vi "诊断标定3.vi"(8 "CAN端口":u16(ring), 9 "设备索引号":u16(ring), 10 "CAN卡类型":u32(ring)=21) -> ()   [LabVIEW 2013] (continued)
                                n480 = call "表格编辑(版本读取).vi"("新元素/子数组"=w689, "活动单元格:单元格背景色"=u32 6618880, "MCListbox引用句柄"=w690) -> ()  [unwired: 1 in, 8 out]
                                }
                                frame 3 {
                                n481 = Index Array(array=w720, index #1=0 ("索引"), index #2=1 ("索引")) -> (element #1=w716:u8, element #2=w717:u8)
                                n482 = Join Numbers(hi=w716, lo=w717) -> ((hi.lo)=w715:u16)
                                n483 = case shown="99, 默认" w715 {
                                tunnel: w720 -> [w723 _ w757]
                                tunnel: w715 -> [_ _ w735]
                                frame 0 {
                                n484 = Index Array(array=w723, index #1=2 ("索引"), index #2=3 ("索引")) -> (element #1=w727:u8, element #2=w726:u8)
                                n485 = Join Numbers(hi=w727, lo=w726) -> ((hi.lo)=w722:u16)
                                n486 = for {
                                N: w722 -> [_]
                                tunnel: w723 -> [w732]
                                tunnel: [w728] -> w721 mode=indexing
                                i -> [w731]
                                n487 = Add(x=w731, y=4) -> (x+y=w729:i32)
                                n488 = Index Array(array=w732, index=w729) -> (element=w728:u8)
                                }
                                "MODEL号" <- w721
                                }
                                frame 99, Default {
                                }
                                frame 1..40 {
                                w740 = ""
                                w761 = "." ("字符串")
                                n489 = Array Subset(array=w757, index=2 ("索引"), length=14 ("长度")) -> (w746:u8[])
                                n490 = Index Array(array=w757, index=16 ("索引")) -> (element=w769:u8)
                                n491 = Index Array(array=w757, index #1=17 ("索引"), index #2=18 ("索引")) -> (element #1=w775:u8, element #2=w776:u8)
                                n492 = Index Array(array=w757, index #1=19 ("索引"), index #2=20 ("索引")) -> (element #1=w770:u8, element #2=w771:u8)
                                n493 = Join Numbers(hi=w770, lo=w771) -> ((hi.lo)=w767:u16)
                                n494 = Join Numbers(hi=w775, lo=w776) -> ((hi.lo)=w768:u16)
                                n495 = Number To Decimal String(number=w735) -> (decimal integer string=w755:string)  [unwired: 1 out]
                                n496 = Number To Decimal String(number=w769) -> (decimal integer string=w763:string)  [unwired: 1 out]
                                n497 = call "数组去零.vi"("输入"=w746) -> ("输出"=w745:dbl[])
                                n498 = Number To Decimal String(number=w768) -> (decimal integer string=w762:string)  [unwired: 1 out]
                                n499 = Number To Decimal String(number=w767) -> (decimal integer string=w760:string)  [unwired: 1 out]
                                n500 = Byte Array To String(unsigned byte array=w745) -> (string=w747:string)
                                n501 = Concatenate Strings("第" ("读取结果"), w755, "模块" ("字符串"), "     读取完成" ("读取结果")) -> (w748:string)
                                n502 = Concatenate Strings("V" ("字符串"), w763, w761, w762, w761, w760) -> (w758:string)
                                n503 = control-ref of="结果"() -> (w751:refnum<vi>)
                                n504 = Array Subset(array=w757, index=23 ("索引"), length=7 ("长度")) -> (w744:u8[])
                                n505 = call "数组去零.vi"("输入"=w744) -> ("输出"=w739:dbl[])
                                n506 = Byte Array To String(unsigned byte array=w739) -> (string=w736:string)
                                n507 = Build Array(w748) -> (w750:string[])
                                n508 = control-ref of="模块软件版本 2"() -> (w752:refnum<vi>)
                                n509 = local read "模块软件版本"() -> (w753:T1)
                                n510 = Equal?(x=w740, y=w736) -> (x = y?=w741:bool)
                                n511 = call "表格编辑(版本读取).vi"("新元素/子数组"=w750, "活动单元格:单元格背景色"=u32 6618880, "MCListbox引用句柄"=w751) -> ()  [unwired: 1 in, 8 out]
                                n512 = Concatenate Strings("-" ("字符串"), w736) -> (w742:string)
                                n513 = Select(t=w740, s=w741, f=w742) -> (s? t:f=w738:string)
                                n514 = Concatenate Strings(w747, "-" ("字符串"), w758, w738) -> (w737:string)
                                n515 = case shown="30" w735 {
                                tunnel: [_ "VERSIONM" "BCUMCAL" "BMUMCAL" "BMURMCAL" "BCUCMCAL" "BCUDMCAL" "SCH" "BSW" "CDD" "DATALAYER" "DATAANALYSIS" "SOC" "SOH" "SOF" "INTRES" "INTCAN" "CARCAN" "CHGCANL" "THM" "CHGM" "HVM" "LVM" "BALM" "SAFEM" "RUNMODEM" "RELAY" "DO" "GBCHGDET" "SUPPLYPOWGDET" "SUMVDET" "CURDET" "TEMPERDET" "CELLVDET" "ISODET" "AI" "DI" "SYSCONF" "ECUCONF"] -> w734
                                frame 0, Default {
                                }
                                frame 1 {
                                }
                                frame 2 {
                                }
                                frame 3 {
                                }
                                frame 4 {
                                }
                                frame 5 {
                                }
                                frame 6 {
                                }
                                frame 7 {
                                }
                                frame 8 {
                                }
                                frame 9 {
                                }
                                frame 10 {
                                }
                                frame 11 {
                                }
                                frame 12 {
                                }
                                frame 13 {
                                }
                                frame 14 {
                                }
                                frame 15 {
                                }
                                frame 16 {
                                }
                                frame 17 {
                                }
                                frame 18 {
                                }
                                frame 19 {
                                }
                                frame 20 {
                                }
                                frame 21 {
                                }
                                frame 22 {
                                }
                                frame 23 {
                                }
                                frame 24 {
                                }
                                frame 25 {
                                }
                                frame 26 {
                                }
                                frame 27 {
                                }
                                frame 28 {
                                }
                                frame 29 {
                                }
                                frame 30 {
                                }
                                frame 31 {
                                }
                                frame 32 {
                                }
                                frame 33 {
                                }
                                frame 34 {
                                }
                                frame 35 {
                                }
                                frame 36 {
                                }
                                frame 37 {
                                }
                                frame 38 {
                                }
                                }
                                n516 = case shown="\"全部读取\"" w753 {
                                tunnel: w737 -> [w820 w828]
                                tunnel: w735 -> [w824 w833]
                                tunnel: w752 -> [w826 w834]
                                tunnel: w734 -> [w825 w832]
                                frame "全部读取" {
                                n517 = Number To Decimal String(number=w824) -> (decimal integer string=w823:string)  [unwired: 1 out]
                                n518 = Concatenate Strings(w823, "-" ("元素"), w825) -> (w821:string)
                                n519 = Build Array(w821, w820) -> (w819:string[])
                                n520 = call "表格编辑(模块版本).vi"("新元素/子数组"=w819, "MCListbox引用句柄"=w826) -> ()  [unwired: 1 in, 9 out]
                                }
                                frame "BCUMCAL", Default {
                                n521 = Number To Decimal String(number=w833) -> (decimal integer string=w831:string)  [unwired: 1 out]
                                n522 = Concatenate Strings(w831, "-" ("元素"), w832) -> (w829:string)
                                n523 = Build Array(w829, w828) -> (w827:string[])
                                n524 = call "表格编辑(模块版本).vi"("新元素/子数组"=w827, "MCListbox引用句柄"=w834) -> ()  [unwired: 1 in, 9 out]
                                }
                                }
                                }
                                }
                                }
                                frame 4 {
                                n525 = Array Subset(array=w847, length=12 ("长度")) -> (w845:u8[])  [unwired: 1 in]
                                n526 = Byte Array To String(unsigned byte array=w845) -> (string=w844:string)
                                n527 = call <vilib>:"Trim Whitespace.vi"("string"=w844) -> ("trimmed string"=w836:string)  [unwired: 1 in]
                                n528 = local read "从板板号"() -> (w835:u8)
                                n529 = local write "硬件版本号"(w836) -> ()
                                n530 = local read "硬件版本"() -> (w837:string[])
                                n531 = Replace Array Subset(array=w837, new element=w836, index=w835) -> (w838:string[])
                                n532 = local write "硬件版本"(w838) -> ()
                                n533 = global write "EV05全局变量1.vi" "写入超时"(TRUE ("写入超时")) -> ()
                                n534 = control-ref of="结果"() -> (w842:refnum<vi>)
                                n535 = Build Array("硬件版本     读取完成" ("读取结果")) -> (w841:string[])
                                n536 = call "表格编辑(版本读取).vi"("新元素/子数组"=w841, "活动单元格:单元格背景色"=u32 6618880, "MCListbox引用句柄"=w842) -> ()  [unwired: 9 out]
                                }
                              }
                              n537 = global write "EV05全局变量1.vi" "写入超时"(TRUE ("写入超时")) -> ()
                            }
                          }
                        }
                        frame True {
                          n538 = Index Array(array=w849, index #1=0 ("索引"), index #2=1 ("索引")) -> (element #1=w854:u8, element #2=w855:u8)
                          n539 = Join Numbers(hi=w854, lo=w855) -> ((hi.lo)=w853:u16)
                          n540 = Number To Hexadecimal String(2:w853) -> (0:w852:string)  [unwired: 1 out]
                          n541 = control-ref of="结果"() -> (w851:refnum<vi>)
                          n542 = Concatenate Strings("0x" ("字符串"), w852) -> (w859:string)
                          n543 = Build Array(w859) -> (w850:string[])
                          n544 = call "表格编辑(版本读取).vi"("新元素/子数组"=w850, "活动单元格:单元格背景色"=u32 16740749, "MCListbox引用句柄"=w851) -> ()  [unwired: 9 out]
                        }
                      }
                      n545 = global write "EV05全局变量1.vi" "流控帧 2"(FALSE ("流控帧 2")) -> ()
                      n546 = local write "控制1"(FALSE ("控制1")) -> ()
                      n547 = local write "消除"(FALSE ("消除")) -> ()
                      n548 = call <vilib>:"Unset Busy.vi"() -> ()  [unwired: 2 in, 10 out]
                    }
                  }
                }
                frame "其它诊断" {
                  n549 = local read "命令序号"() -> (w861:u8)
                  n550 = call "多帧接收机制(EV05).vi"("can卡类型"=w868, "设备索引号"=w867, "CAN端口"=w866, "VCI_Receive"=w865, "命令"=w863, "板号"=w864, "命令序号"=w861) -> ("错误代码"=w870:i32, "输出数组"=w862:u8[], "读错误代码"=w860:u8[], "结束信号"=w869:bool)  [unwired: 1 in, 8 out]
                  n551 = case shown="真" w869 {
                    tunnel: w871 -> [_ w872]
                    tunnel: w870 -> [_ _]
                    tunnel: w862 -> [_ w873]
                    tunnel: w861 -> [_ w876]
                    tunnel: w860 -> [_ w874]
                    frame False {
                    }
                    frame True {
                      n552 = Insert Into Array(array=w874, new element=w873) -> (w875:u8[])  [unwired: 1 in]
                      n553 = case shown="1" w876 {
                        tunnel: w875 -> [_ w885 w971]
                        tunnel: w872 -> [_ _ w966]
                        frame 0, Default {
                        }
                        frame 1 {
                          n554 = Index Array(array=w885) -> (element #1=w884:u8, element #2=w883:u8, element #3=w882:u8)  [unwired: 3 in]
                          n555 = Join Numbers(hi=w883, lo=w882) -> ((hi.lo)=w881:u16)
                          n556 = case shown="4" w884 {
                            tunnel: w885 -> [_ _ _ _ _ _ _ _ _ _]
                            tunnel: w881 -> [_ w888 w896 w906 w916 w926 w936 w946 w956 _]
                            frame 0, Default {
                              n557 = local write "继电器超时处理"(FALSE ("继电器超时处理")) -> ()
                            }
                            frame 1 {
                              n558 = Equal To 0?(x=w888) -> (x = 0?=w887:bool)
                              n559 = local write "正级继电器 12"(w887) -> ()
                              n560 = case shown="假" w887 {
                                tunnel: w888 -> [w891 _]
                                frame False {
                                n561 = local read "正级继电器"() -> (w893:bool)
                                n562 = Number To Hexadecimal String(2:w891) -> (0:w890:string)  [unwired: 1 out]
                                n563 = local write "继电器超时处理"(TRUE ("继电器超时处理")) -> ()
                                n564 = Not(x=w893) -> (.not. x?=w892:bool)
                                n565 = Concatenate Strings("继电器操作失败,0x" ("消息"), w890) -> ()  [unwired: 1 out]
                                n566 = local write "正级继电器"(w892) -> ()
                                }
                                frame True {
                                (unwired) "继电器操作成功!\n继电器操作成功!\n继电器操作成功!"
                                }
                              }
                            }
                            frame 2 {
                              n567 = Equal To 0?(x=w896) -> (x = 0?=w895:bool)
                              n568 = case shown="假" w895 {
                                tunnel: w896 -> [w902 _]
                                tunnel: [w900 "继电器操作成功!\n继电器操作成功!\n继电器操作成功!"] -> _
                                frame False {
                                n569 = local read "负级继电器"() -> (w898:bool)
                                n570 = Number To Hexadecimal String(2:w902) -> (0:w901:string)  [unwired: 1 out]
                                n571 = local write "继电器超时处理"(TRUE ("继电器超时处理")) -> ()
                                n572 = Not(x=w898) -> (.not. x?=w899:bool)
                                n573 = Concatenate Strings("继电器操作失败,0x" ("消息"), w901) -> (w900:string)
                                n574 = local write "负级继电器"(w899) -> ()
                                }
                                frame True {
                                }
                              }
                              n575 = local write "正级继电器 2"(w895) -> ()
                            }
                            frame 3 {
                              n576 = Equal To 0?(x=w906) -> (x = 0?=w905:bool)
                              n577 = case shown="假" w905 {
                                tunnel: w906 -> [w912 _]
                                tunnel: [w910 "继电器操作成功!\n继电器操作成功!\n继电器操作成功!"] -> _
                                frame False {
                                n578 = local read "预充电继电器"() -> (w908:bool)
                                n579 = Number To Hexadecimal String(2:w912) -> (0:w911:string)  [unwired: 1 out]
                                n580 = local write "继电器超时处理"(TRUE ("继电器超时处理")) -> ()
                                n581 = Not(x=w908) -> (.not. x?=w909:bool)
                                n582 = Concatenate Strings("继电器操作失败,0x" ("消息"), w911) -> (w910:string)
                                n583 = local write "预充电继电器"(w909) -> ()
                                }
                                frame True {
                                }
                              }
                              n584 = local write "正级继电器 3"(w905) -> ()
                            }
                            frame 4 {
                              n585 = Equal To 0?(x=w916) -> (x = 0?=w915:bool)
                              n586 = case shown="假" w915 {
                                tunnel: w916 -> [w922 _]
                                tunnel: [w920 "继电器操作成功!\n继电器操作成功!\n继电器操作成功!"] -> _
                                frame False {
                                n587 = local read "加热继电器"() -> (w919:bool)
                                n588 = Number To Hexadecimal String(2:w922) -> (0:w921:string)  [unwired: 1 out]
                                n589 = local write "继电器超时处理"(TRUE ("继电器超时处理")) -> ()
                                n590 = Not(x=w919) -> (.not. x?=w918:bool)
                                n591 = Concatenate Strings("继电器操作失败,0x" ("消息"), w921) -> (w920:string)
                                n592 = local write "加热继电器"(w918) -> ()
                                }
                                frame True {
                                }
                              }
                              n593 = local write "正级继电器 5"(w915) -> ()
                            }
                            frame 5 {
                              n594 = Equal To 0?(x=w926) -> (x = 0?=w925:bool)
                              n595 = case shown="假" w925 {
                                tunnel: w926 -> [w932 _]
                                tunnel: [w930 "继电器操作成功!\n继电器操作成功!\n继电器操作成功!"] -> _
                                frame False {
                                n596 = local read "充电继电器"() -> (w928:bool)
                                n597 = Number To Hexadecimal String(2:w932) -> (0:w931:string)  [unwired: 1 out]
                                n598 = local write "继电器超时处理"(TRUE ("继电器超时处理")) -> ()
                                n599 = Not(x=w928) -> (.not. x?=w929:bool)
                                n600 = Concatenate Strings("继电器操作失败,0x" ("消息"), w931) -> (w930:string)
                                n601 = local write "充电继电器"(w929) -> ()
                                }
                                frame True {
                                }
                              }
                              n602 = local write "正级继电器 4"(w925) -> ()
                            }
                            frame 6 {
                              n603 = Equal To 0?(x=w936) -> (x = 0?=w935:bool)
                              n604 = local write "正级继电器 6"(w935) -> ()
                              n605 = case shown="假" w935 {
                                tunnel: w936 -> [w942 _]
                                tunnel: [w940 "继电器操作成功!\n继电器操作成功!\n继电器操作成功!"] -> _
                                frame False {
                                n606 = local read "风机继电器"() -> (w938:bool)
                                n607 = Number To Hexadecimal String(2:w942) -> (0:w941:string)  [unwired: 1 out]
                                n608 = local write "继电器超时处理"(TRUE ("继电器超时处理")) -> ()
                                n609 = Not(x=w938) -> (.not. x?=w939:bool)
                                n610 = Concatenate Strings("继电器操作失败,0x" ("消息"), w941) -> (w940:string)
                                n611 = local write "风机继电器"(w939) -> ()
                                }
                                frame True {
                                }
                              }
                            }
                            frame 7 {
                              n612 = Equal To 0?(x=w946) -> (x = 0?=w945:bool)
                              n613 = case shown="假" w945 {
                                tunnel: w946 -> [w951 _]
                                tunnel: [w949 "继电器操作成功!\n继电器操作成功!\n继电器操作成功!"] -> _
                                frame False {
                                n614 = local read "加热继电器(从)"() -> (w947:bool)
                                n615 = Number To Hexadecimal String(2:w951) -> (0:w950:string)  [unwired: 1 out]
                                n616 = Not(x=w947) -> (.not. x?=w948:bool)
                                n617 = Concatenate Strings("继电器操作失败,0x" ("消息"), w950) -> (w949:string)
                                n618 = local write "加热继电器(从)"(w948) -> ()
                                }
                                frame True {
                                n619 = local write "继电器超时处理"(TRUE ("继电器超时处理")) -> ()
                                }
                              }
                              n620 = local write "正级继电器 7"(w945) -> ()
                            }
                            frame 8 {
                              n621 = Equal To 0?(x=w956) -> (x = 0?=w955:bool)
                              n622 = case shown="假" w955 {
                                tunnel: w956 -> [w961 _]
                                tunnel: [w959 "继电器操作成功!\n继电器操作成功!\n继电器操作成功!"] -> _
                                frame False {
                                n623 = local read "风机继电器(从)"() -> (w957:bool)
                                n624 = Number To Hexadecimal String(2:w961) -> (0:w960:string)  [unwired: 1 out]
                                n625 = Not(x=w957) -> (.not. x?=w958:bool)
                                n626 = Concatenate Strings("继电器操作失败,0x" ("消息"), w960) -> (w959:string)
                                n627 = local write "风机继电器(从)"(w958) -> ()
                                }
                                frame True {
                                n628 = local write "继电器超时处理"(TRUE ("继电器超时处理")) -> ()
                                }
                              }
                              n629 = local write "正级继电器 8"(w955) -> ()
                            }
                            frame 85, 170 {
                              n630 = local write "继电器超时处理"(TRUE ("继电器超时处理")) -> ()
                            }
                          }
                        }
                        frame 2 {
                          n631 = Index Array(array=w971) -> (element #1=w970:u8, element #2=w969:u8, element #3=w968:u8)  [unwired: 3 in]
                          n632 = Join Numbers(hi=w969, lo=w968) -> ((hi.lo)=w967:u16)
                          n633 = case shown="2" w970 {
                            tunnel: w971 -> [_ _ _]
                            tunnel: w967 -> [_ w975 w989]
                            tunnel: w966 -> [_ w974 _]
                            frame 0, Default {
                              n634 = local write "继电器超时处理"(FALSE ("继电器超时处理")) -> ()
                            }
                            frame 1 {
                              n635 = Equal To 0?(x=w975) -> (x = 0?=w973:bool)
                              n636 = case shown="假" w973 {
                                tunnel: w975 -> [w981 _]
                                tunnel: [w979 "DO控制操作成功!\nDO控制操作成功!\nDO控制操作成功!"] -> _
                                tunnel: w974 -> [w978 _]
                                frame False {
                                n637 = case shown="\"主板\", 默认" w978 {
                                frame "主板", Default {
                                n638 = local read "DO1"() -> (w984:bool)
                                n639 = Not(x=w984) -> (.not. x?=w983:bool)
                                n640 = local write "DO1"(w983) -> ()
                                }
                                frame "从板" {
                                n641 = local read "DO1 2"() -> (w986:bool)
                                n642 = Not(x=w986) -> (.not. x?=w985:bool)
                                n643 = local write "DO1 2"(w985) -> ()
                                }
                                }
                                n644 = Number To Hexadecimal String(2:w981) -> (0:w980:string)  [unwired: 1 out]
                                n645 = Concatenate Strings("DO控制操作失败,0x" ("消息"), w980) -> (w979:string)
                                }
                                frame True {
                                }
                              }
                              n646 = case shown="\"从板\"" w974 {
                                tunnel: w973 -> [w976 w977]
                                frame "主板", Default {
                                n647 = local write "正级继电器 9"(w976) -> ()
                                }
                                frame "从板" {
                                n648 = local write "正级继电器 11"(w977) -> ()
                                }
                              }
                            }
                            frame 2 {
                              n649 = Equal To 0?(x=w989) -> (x = 0?=w988:bool)
                              n650 = case shown="假" w988 {
                                tunnel: w989 -> [w994 _]
                                tunnel: [w992 "DO控制操作成功!\nDO控制操作成功!\nDO控制操作成功!"] -> _
                                frame False {
                                n651 = Number To Hexadecimal String(2:w994) -> (0:w993:string)  [unwired: 1 out]
                                n652 = local read "DO2"() -> (w991:bool)
                                n653 = Not(x=w991) -> (.not. x?=w990:bool)
                                n654 = Concatenate Strings("DO控制操作失败,0x" ("消息"), w993) -> (w992:string)
                                n655 = local write "DO2"(w990) -> ()
                                }
                                frame True {
                                }
                              }
                              n656 = local write "正级继电器 10"(w988) -> ()
                            }
                          }
                        }
                      }
                      n657 = local write "消除"(FALSE ("消除")) -> ()
                      n658 = global write "EV05全局变量1.vi" "流控帧 2"(FALSE ("流控帧 2")) -> ()
                      n659 = local write "控制1"(FALSE ("控制1")) -> ()
                      "继电器超时处理" <- TRUE ("控制1")
                    }
                  }
                }
                frame "高压板校正" {
                  n660 = local read "命令序号"() -> (w1001:u8)
                  n661 = call "多帧接收机制(EV05).vi"("can卡类型"=w1008, "设备索引号"=w1007, "CAN端口"=w1006, "VCI_Receive"=w1005, "命令"=w1003, "板号"=w1004, "命令序号"=w1001) -> ("错误信号"=w997:bool, "错误代码"=w1010:i32, "输出数组"=w1002:u8[], "读错误代码"=w1000:u8[], "结束信号"=w1009:bool)  [unwired: 1 in, 7 out]
                  n662 = local read "控制1"() -> (w998:bool)
                  n663 = And(x=w998, y=w1009) -> (x .and. y?=w999:bool)
                  n664 = case shown="真" w999 {
                    tunnel: w1011 -> [_ w1015]
                    tunnel: w1010 -> [_ _]
                    tunnel: w1002 -> [_ w1013]
                    tunnel: w1001 -> [_ w1014]
                    tunnel: w1000 -> [_ w1016]
                    tunnel: w997 -> [_ w1017]
                    frame False {
                    }
                    frame True {
                      n665 = case shown="假" w1017 {
                        tunnel: w1016 -> [_ w1227]
                        tunnel: w1015 -> [_ _]
                        tunnel: w1014 -> [w1022 _]
                        tunnel: w1013 -> [w1021 _]
                        frame False {
                          n666 = case shown="2" w1022 {
                            tunnel: w1021 -> [_ w1027 w1061 w1091 w1118 w1145 w1172 w1199]
                            frame 0, Default {
                            }
                            frame 1 {
                              n667 = for {
                                N: 10 -> [_]
                                tunnel: w1027 -> [w1044]
                                shift-right: [w1031] -> w1025
                                shift-left: string[] [] -> [w1033]
                                i -> [w1030]
                                w1038 = 8 ("索引")
                                w1042 = 2 ("y")
                                n668 = Multiply(x=w1030, y=w1042) -> (x*y=w1043:i32)
                                n669 = Array Subset(array=w1044, index=w1043, length=w1042) -> (w1041:u8[])
                                n670 = Index Array(array=w1041) -> (element #1=w1040:u8, element #2=w1039:u8)  [unwired: 2 in]
                                n671 = call "二进制解析-8.6.vi"("索引"=w1038, "数值"=w1040) -> ("低位子数组"=w1037:i32[])  [unwired: 1 in, 2 out]
                                n672 = call "二进制解析-8.6.vi"("索引"=w1038, "数值"=w1039) -> ("低位子数组"=w1036:i32[])  [unwired: 1 in, 2 out]
                                n673 = Insert Into Array(array=w1037, new element=w1036) -> (w1035:i32[])  [unwired: 1 in]
                                n674 = case shown="2" w1030 {
                                tunnel: [6 15 9 4 2 0 2] -> w1029
                                frame 0, Default {
                                }
                                frame 1 {
                                }
                                frame 2 {
                                }
                                frame 3..5 {
                                }
                                frame 8, 9 {
                                }
                                frame 7 {
                                }
                                frame 6 {
                                }
                                }
                                n675 = Reverse 1D Array(array=w1035) -> (reversed array=w1034:i32[])
                                n676 = for {
                                N: w1029 -> [_]
                                tunnel: w1034 -> [w1056] mode=indexing
                                tunnel: [w1052] -> w1032 mode=indexing
                                n677 = Equal To 0?(x=w1056) -> (x = 0?=w1055:bool)
                                n678 = Select(t="无", s=w1055, f="故障") -> (s? t:f=w1052:string)
                                }
                                n679 = Insert Into Array(array=w1033, new element=w1032) -> (w1031:string[])  [unwired: 1 in]
                              }
                              n680 = call "详细故障分解.vi"("名称"=string[] ["上电自检异常(CellV)", "通讯异常(CellV)", "不更新(CellV)", "未校准(CellV)", "保留", "采样线路断路(CellV)", "18b20上电自检异常(T) ", "18b20通讯异常(T)", "18b20传感器丢失(T)", "18b20传感器无号(T)", "18b20温度异常跳变(T)", "18b20信号线对电源短路(T)", "18b20信号线对地短路(T)", "18b20 CRC校验异常(T)", "NTC上电自检异常(T)", "NTC通讯异常(T)", "NTC传感器丢失(T)", "NTC温度异常跳变(T)", "NTC信号线断路(T)", "NTC信号线对电源短(T)", "NTC信号线对地短路(T)", "上电自检异常(Curr)", "参数异常(Curr)", "不更新(Curr)", "未校准(Curr)", "采样线断开(Curr)", "电流零漂异常(Curr)", "传感器反接(Curr)", "读取实时电流故障(Curr)", "平均电流故障(Curr)", "自检异常(iso)", "前端检测电阻损坏(iso)", "不更新(iso)", "未校准(iso)", "上电自检异常(Sumv_in)", "通讯异常(Sumv_in)", "不更新(Sumv_in)", "未校准(Sumv_in)", "上电自检异常(Sumv_out)", "通讯异常(Sumv_out)", "不更新(Sumv_out)", "未校准(Sumv_out)", "系统时钟自检异常(Clock)", "系统时钟未校准(Clock)", "充电均衡模块不能开启", "充电均衡模块不能关闭", "放电均衡模块不能开启", "放电均衡模块不能关闭"], "故障输入口"=w1025) -> ("输出数组"=w1023:string[][])  [unwired: 1 in, 2 out]
                              n681 = local write "电池故障"(w1023) -> ()
                            }
                            frame 2 {
                              n682 = for {
                                N: 5 -> [_]
                                tunnel: w1061 -> [w1078]
                                shift-right: [w1065] -> w1059
                                shift-left: string[] [] -> [w1067]
                                i -> [w1063]
                                w1072 = 8 ("索引")
                                w1076 = 2 ("y")
                                n683 = Multiply(x=w1063, y=w1076) -> (x*y=w1077:i32)
                                n684 = Array Subset(array=w1078, index=w1077, length=w1076) -> (w1075:u8[])
                                n685 = Index Array(array=w1075) -> (element #1=w1074:u8, element #2=w1073:u8)  [unwired: 2 in]
                                n686 = call "二进制解析-8.6.vi"("索引"=w1072, "数值"=w1074) -> ("低位子数组"=w1071:i32[])  [unwired: 1 in, 2 out]
                                n687 = call "二进制解析-8.6.vi"("索引"=w1072, "数值"=w1073) -> ("低位子数组"=w1070:i32[])  [unwired: 1 in, 2 out]
                                n688 = Insert Into Array(array=w1071, new element=w1070) -> (w1069:i32[])  [unwired: 1 in]
                                n689 = case shown="2" w1063 {
                                tunnel: [4 6 5] -> w1064
                                frame 0, Default {
                                }
                                frame 2 {
                                }
                                frame 4 {
                                }
                                }
                                n690 = Reverse 1D Array(array=w1069) -> (reversed array=w1068:i32[])
                                n691 = for {
                                N: w1064 -> [_]
                                tunnel: w1068 -> [w1086] mode=indexing
                                tunnel: [w1082] -> w1066 mode=indexing
                                n692 = Equal To 0?(x=w1086) -> (x = 0?=w1085:bool)
                                n693 = Select(t="无", s=w1085, f="故障") -> (s? t:f=w1082:string)
                                }
                                n694 = Insert Into Array(array=w1067, new element=w1066) -> (w1065:string[])  [unwired: 1 in]
                              }
                              n695 = call "详细故障分解.vi"("名称"=string[] ["自检异常(ee_cpu)", "存储空间满(ee_cpu)", "数据写入失败(ee_cpu)", "数据读取异常(ee_cpu)", "自检异常(ee_ext)", "存储空间满(ee_ext)", "数据写入失败(ee_ext)", "数据读取异常(ee_ext)", "自检异常(flash_ext)", "故障数据存储空间满(flash_ext)", "历史数据存储空间满(flash_ext)", "数据写入失败(flash_ext)", "数据读取失败(flash_ext)", "数据校验异常(flash_ext)", "自检异常(flash_cpu)", "存储空间满(flash_cpu)", "数据写入失败(flash_cpu)", "数据读取异常(flash_cpu)", "应用程序异常(cpu)", "应用程序下载异常(cpu)", "AD模块异常(cpu)", "RAM异常(cpu)", "CPU异常下电(cpu)"], "故障输入口"=w1059) -> ("输出数组"=w1057:string[][])  [unwired: 1 in, 2 out]
                              n696 = local write "电池故障"(w1057) -> ()
                            }
                            frame 3 {
                              n697 = for {
                                N: 5 -> [_]
                                tunnel: w1091 -> [w1108]
                                shift-right: [w1095] -> w1089
                                shift-left: string[] [] -> [w1097]
                                i -> [w1094]
                                w1102 = 8 ("索引")
                                w1106 = 2 ("y")
                                n698 = Multiply(x=w1094, y=w1106) -> (x*y=w1107:i32)
                                n699 = Array Subset(array=w1108, index=w1107, length=w1106) -> (w1105:u8[])
                                n700 = Index Array(array=w1105) -> (element #1=w1104:u8, element #2=w1103:u8)  [unwired: 2 in]
                                n701 = call "二进制解析-8.6.vi"("索引"=w1102, "数值"=w1104) -> ("低位子数组"=w1101:i32[])  [unwired: 1 in, 2 out]
                                n702 = call "二进制解析-8.6.vi"("索引"=w1102, "数值"=w1103) -> ("低位子数组"=w1100:i32[])  [unwired: 1 in, 2 out]
                                n703 = Insert Into Array(array=w1101, new element=w1100) -> (w1099:i32[])  [unwired: 1 in]
                                n704 = Reverse 1D Array(array=w1099) -> (reversed array=w1098:i32[])
                                n705 = for {
                                N: 6 -> [_]
                                tunnel: w1098 -> [w1113] mode=indexing
                                tunnel: [w1109] -> w1096 mode=indexing
                                n706 = Equal To 0?(x=w1113) -> (x = 0?=w1112:bool)
                                n707 = Select(t="无", s=w1112, f="故障") -> (s? t:f=w1109:string)
                                }
                                n708 = Insert Into Array(array=w1097, new element=w1096) -> (w1095:string[])  [unwired: 1 in]
                              }
                              n709 = call "详细故障分解.vi"("名称"=string[] ["初始化失败(CAN4)", "发送异常(CAN4)", "接收异常(CAN4)", "总线超时(CAN4)", "BUSOFF(CAN4)", "帧格式(CAN4)", "初始化异常(CAN0)", "发送异常(CAN0)", "接收异常(CAN0)", "总线超时(CAN0)", "BUSOFF(CAN0)", "帧格式(CAN0)", "初始化异常(CAN1)", "发送异常(CAN1)", "接收异常(CAN1)", "总线超时(CAN1)", "BUSOFF(CAN1)", "帧格式(CAN1)", "初始化失败(CAN2)", "发送异常(CAN2)", "接收异常(CAN2)", "总线超时(CAN2)", "BUSOFF(CAN2)", "帧格式(CAN2)", "初始化失败(CAN3)", "发送异常(CAN3)", "接收异常(CAN3)", "总线超时(CAN3)", "BUSOFF(CAN3)", "帧格式(CAN3)"], "故障输入口"=w1089) -> ("输出数组"=w1087:string[][])  [unwired: 1 in, 2 out]
                              n710 = local write "电池故障"(w1087) -> ()
                            }
                            frame 4 {
                              n711 = for {
                                N: 1 -> [_]
                                tunnel: w1118 -> [w1135]
                                shift-right: [w1122] -> w1116
                                shift-left: string[] [] -> [w1124]
                                i -> [w1121]
                                w1129 = 8 ("索引")
                                w1133 = 2 ("y")
                                n712 = Multiply(x=w1121, y=w1133) -> (x*y=w1134:i32)
                                n713 = Array Subset(array=w1135, index=w1134, length=w1133) -> (w1132:u8[])
                                n714 = Index Array(array=w1132) -> (element #1=w1131:u8, element #2=w1130:u8)  [unwired: 2 in]
                                n715 = call "二进制解析-8.6.vi"("索引"=w1129, "数值"=w1131) -> ("低位子数组"=w1128:i32[])  [unwired: 1 in, 2 out]
                                n716 = call "二进制解析-8.6.vi"("索引"=w1129, "数值"=w1130) -> ("低位子数组"=w1127:i32[])  [unwired: 1 in, 2 out]
                                n717 = Insert Into Array(array=w1128, new element=w1127) -> (w1126:i32[])  [unwired: 1 in]
                                n718 = Reverse 1D Array(array=w1126) -> (reversed array=w1125:i32[])
                                n719 = for {
                                N: 4 -> [_]
                                tunnel: w1125 -> [w1140] mode=indexing
                                tunnel: [w1136] -> w1123 mode=indexing
                                n720 = Equal To 0?(x=w1140) -> (x = 0?=w1139:bool)
                                n721 = Select(t="无", s=w1139, f="故障") -> (s? t:f=w1136:string)
                                }
                                n722 = Insert Into Array(array=w1124, new element=w1123) -> (w1122:string[])  [unwired: 1 in]
                              }
                              n723 = call "详细故障分解.vi"("名称"=string[] ["通讯协议版本不一致(soft)", "系统不同步(soft)", "软件版本不一致(soft)", "同硬件平台不兼容(soft)"], "故障输入口"=w1116) -> ("输出数组"=w1114:string[][])  [unwired: 1 in, 2 out]
                              n724 = local write "电池故障"(w1114) -> ()
                            }
                            frame 5 {
                              n725 = for {
                                N: 2 -> [_]
                                tunnel: w1145 -> [w1162]
                                shift-right: [w1149] -> w1143
                                shift-left: string[] [] -> [w1151]
                                i -> [w1148]
                                w1156 = 8 ("索引")
                                w1160 = 2 ("y")
                                n726 = Multiply(x=w1148, y=w1160) -> (x*y=w1161:i32)
                                n727 = Array Subset(array=w1162, index=w1161, length=w1160) -> (w1159:u8[])
                                n728 = Index Array(array=w1159) -> (element #1=w1158:u8, element #2=w1157:u8)  [unwired: 2 in]
                                n729 = call "二进制解析-8.6.vi"("索引"=w1156, "数值"=w1158) -> ("低位子数组"=w1155:i32[])  [unwired: 1 in, 2 out]
                                n730 = call "二进制解析-8.6.vi"("索引"=w1156, "数值"=w1157) -> ("低位子数组"=w1154:i32[])  [unwired: 1 in, 2 out]
                                n731 = Insert Into Array(array=w1155, new element=w1154) -> (w1153:i32[])  [unwired: 1 in]
                                n732 = Reverse 1D Array(array=w1153) -> (reversed array=w1152:i32[])
                                n733 = for {
                                N: 4 -> [_]
                                tunnel: w1152 -> [w1167] mode=indexing
                                tunnel: [w1163] -> w1150 mode=indexing
                                n734 = Equal To 0?(x=w1167) -> (x = 0?=w1166:bool)
                                n735 = Select(t="无", s=w1166, f="故障") -> (s? t:f=w1163:string)
                                }
                                n736 = Insert Into Array(array=w1151, new element=w1150) -> (w1149:string[])  [unwired: 1 in]
                              }
                              n737 = call "详细故障分解.vi"("名称"=string[] ["初始化失败(RS232)", "发送异常(RS232)", "接收异常(RS232)", "总线超时(RS232)", "初始化失败(RS485)", "发送异常(RS485)", "接收异常(RS485)", "总线超时(RS485)"], "故障输入口"=w1143) -> ("输出数组"=w1141:string[][])  [unwired: 1 in, 2 out]
                              n738 = local write "电池故障"(w1141) -> ()
                            }
                            frame 6 {
                              n739 = for {
                                N: 2 -> [_]
                                tunnel: w1172 -> [w1189]
                                shift-right: [w1176] -> w1170
                                shift-left: string[] [] -> [w1178]
                                i -> [w1175]
                                w1183 = 8 ("索引")
                                w1187 = 2 ("y")
                                n740 = Multiply(x=w1175, y=w1187) -> (x*y=w1188:i32)
                                n741 = Array Subset(array=w1189, index=w1188, length=w1187) -> (w1186:u8[])
                                n742 = Index Array(array=w1186) -> (element #1=w1185:u8, element #2=w1184:u8)  [unwired: 2 in]
                                n743 = call "二进制解析-8.6.vi"("索引"=w1183, "数值"=w1185) -> ("低位子数组"=w1182:i32[])  [unwired: 1 in, 2 out]
                                n744 = call "二进制解析-8.6.vi"("索引"=w1183, "数值"=w1184) -> ("低位子数组"=w1181:i32[])  [unwired: 1 in, 2 out]
                                n745 = Insert Into Array(array=w1182, new element=w1181) -> (w1180:i32[])  [unwired: 1 in]
                                n746 = Reverse 1D Array(array=w1180) -> (reversed array=w1179:i32[])
                                n747 = for {
                                N: 16 -> [_]
                                tunnel: w1179 -> [w1194] mode=indexing
                                tunnel: [w1190] -> w1177 mode=indexing
                                n748 = Equal To 0?(x=w1194) -> (x = 0?=w1193:bool)
                                n749 = Select(t="无", s=w1193, f="故障") -> (s? t:f=w1190:string)
                                }
                                n750 = Insert Into Array(array=w1178, new element=w1177) -> (w1176:string[])  [unwired: 1 in]
                              }
                              n751 = call "详细故障分解.vi"("名称"=string[] ["DI1对地短", "DI1对电源短", "DI2对地短", "DI2对电源短", "DI3对地短", "DI3对电源短", "DI4对地短", "DI4对电源短", "DI5对地短", "DI5对电源短", "DI6对地短", "DI6对电源短", "DI7对地短", "DI7对电源短", "DI8对地短", "DI8对电源短", "DO1对地短", "DO1对电源短", "DO2对地短", "DO2对电源短", "DO3对地短", "DO3对电源短", "DO4对地短", "DO4对电源短", "DO5对地短", "DO5对电源短", "DO6对地短", "DO6对电源短", "DO7对地短", "DO7对电源短", "DO8对地短", "DO8对电源短"], "故障输入口"=w1170) -> ("输出数组"=w1168:string[][])  [unwired: 1 in, 2 out]
                              n752 = local write "电池故障"(w1168) -> ()
                            }
                            frame 7 {
                              n753 = for {
                                N: 2 -> [_]
                                tunnel: w1199 -> [w1216]
                                shift-right: [w1203] -> w1197
                                shift-left: string[] [] -> [w1205]
                                i -> [w1201]
                                w1210 = 8 ("索引")
                                w1214 = 2 ("y")
                                n754 = Multiply(x=w1201, y=w1214) -> (x*y=w1215:i32)
                                n755 = Array Subset(array=w1216, index=w1215, length=w1214) -> (w1213:u8[])
                                n756 = Index Array(array=w1213) -> (element #1=w1212:u8, element #2=w1211:u8)  [unwired: 2 in]
                                n757 = call "二进制解析-8.6.vi"("索引"=w1210, "数值"=w1212) -> ("低位子数组"=w1209:i32[])  [unwired: 1 in, 2 out]
                                n758 = call "二进制解析-8.6.vi"("索引"=w1210, "数值"=w1211) -> ("低位子数组"=w1208:i32[])  [unwired: 1 in, 2 out]
                                n759 = Insert Into Array(array=w1209, new element=w1208) -> (w1207:i32[])  [unwired: 1 in]
                                n760 = case shown="1" w1201 {
                                tunnel: [4 6] -> w1202
                                frame 0, Default {
                                }
                                frame 1 {
                                }
                                }
                                n761 = Reverse 1D Array(array=w1207) -> (reversed array=w1206:i32[])
                                n762 = for {
                                N: w1202 -> [_]
                                tunnel: w1206 -> [w1223] mode=indexing
                                tunnel: [w1219] -> w1204 mode=indexing
                                n763 = Equal To 0?(x=w1223) -> (x = 0?=w1222:bool)
                                n764 = Select(t="无", s=w1222, f="故障") -> (s? t:f=w1219:string)
                                }
                                n765 = Insert Into Array(array=w1205, new element=w1204) -> (w1203:string[])  [unwired: 1 in]
                              }
                              n766 = call "详细故障分解.vi"("名称"=string[] ["超时(pre-chg)", "后端开路(pre-chg)", "后端短路(pre-chg)", "预充电回路断开(pre-chg)", "正级继电器驱动故障(relay_driver)", "负级继电器驱动故障(relay_driver)", "预充电继电器驱动故障(relay_driver)", "充电继电器驱动故障(relay_driver)", "风机继电器驱动故障(relay_driver)", "加热继电器驱动故障(relay_driver)"], "故障输入口"=w1197) -> ("输出数组"=w1195:string[][])  [unwired: 1 in, 2 out]
                              n767 = local write "电池故障"(w1195) -> ()
                            }
                          }
                        }
                        frame True {
                          n768 = Index Array(array=w1227, index #1=0 ("索引"), index #2=1 ("索引")) -> (element #1=w1230:u8, element #2=w1231:u8)
                          n769 = Join Numbers(hi=w1230, lo=w1231) -> ((hi.lo)=w1229:u16)
                          n770 = Number To Hexadecimal String(2:w1229) -> (0:w1228:string)  [unwired: 1 out]
                          n771 = Concatenate Strings("读取错误，代码： " ("字符串"), "0x" ("字符串"), w1228) -> (w1226:string)
                          n772 = One Button Dialog(message=w1226, button name ("OK")="是" ("按钮名称（“确定”）")) -> ()  [unwired: 1 out]
                        }
                      }
                      n773 = local write "消除"(FALSE ("消除")) -> ()
                      n774 = global write "EV05全局变量1.vi" "流控帧 2"(FALSE ("流控帧 2")) -> ()
                      n775 = local write "控制1"(FALSE ("控制1")) -> ()
                      n776 = global write "EV05全局变量1.vi" "写入超时"(TRUE ("写入超时")) -> ()
                    }
                  }
                }
              }
            }
          }
        }
      }
      frame Error {
      }
    }
  }
  n777 = while {
    tunnel: w36 -> [w1243]
    tunnel: w35 -> [w1242]
    tunnel: [w1241] -> w34
    tunnel: [w1240] -> w33
    tunnel: w23 -> [_]
    tunnel: w20 -> [_]
    stop <- w1239 stop-if-true
    n778 = event shown="[19] \"主界面选项\": 值改变" {
      selector: _ -> [_ _ _ _ _ _ _ _ _ _ _ _ _ _ _ _ _ _ _ _ _ _ _ _ _ _ _ _ _ _ _ _ _ _ _ _ _ _ _ _ _ _ _ _ _ _ _ _ _ _ _ _ _]
      dyn-events: _ -> [_ _ _ _ _ _ _ _ _ _ _ _ _ _ _ _ _ _ _ _ _ _ _ _ _ _ _ _ _ _ _ _ _ _ _ _ _ _ _ _ _ _ _ _ _ _ _ _ _ _ _ _ _]
      timeout: 200 -> [_ _ _ _ _ _ _ _ _ _ _ _ _ _ _ _ _ _ _ _ _ _ _ _ _ _ _ _ _ _ _ _ _ _ _ _ _ _ _ _ _ _ _ _ _ _ _ _ _ _ _ _ _]
      tunnel: [_ w1246 w1286 _ _ _ _ _ _ _ _ _ _ _ _ _ _ _ _ _ _ _ _ _ _ _ _ _ _ _ _ _ _ _ _ _ _ _ _ _ _ _ _ _ _ _ _ _ _ _ _ _ _] -> w1238
      tunnel: w1243 -> [w1245 w1249 w1285 _ w1326 w1337 w1348 w1359 w1370 w1381 w1392 w1403 w1414 w1425 w1436 w1447 w1463 w2001 w2423 w2448 w2476 w2579 w2652 w2665 w2675 w2721 _ _ w2771 w2838 w2905 w2972 w3039 w3106 w3173 w3241 w3309 w3376 w3443 w3513 w3524 w3563 w3603 w3643 w3683 w3721 w3781 w3816 w3852 w3885 w3955 w3988 w4021]
      tunnel: w1242 -> [w1244 w1248 w1284 _ w1325 w1336 w1347 w1358 w1369 w1380 w1391 w1402 w1413 w1424 w1435 w1446 w1462 w2000 w2422 w2447 w2475 w2578 w2650 w2663 w2674 w2720 _ _ w2770 w2837 w2904 w2971 w3038 w3105 w3172 w3240 w3308 w3375 w3442 w3511 w3523 w3562 w3602 w3642 w3682 w3720 w3780 w3815 w3851 w3884 w3954 w3987 w4020]
      tunnel: [w1245 w1249 w1285 _ w1326 w1337 w1348 w1359 w1370 w1381 w1392 w1403 w1414 w1425 w1436 w1447 w1463 w2001 w2423 w2448 w2476 w2579 w2651 w2664 w2675 w2721 _ _ w2771 w2838 w2905 w2972 w3039 w3106 w3173 w3241 w3309 w3376 w3443 w3512 w3522 w3561 w3601 w3641 w3681 w3721 w3779 w3814 w3850 w3883 w3953 w3986 w4019] -> w1241
      tunnel: [w1244 w1248 w1284 _ w1325 w1336 w1347 w1358 w1369 w1380 w1391 w1402 w1413 w1424 w1435 w1446 w1462 w2000 w2422 w2447 w2475 w2578 w2649 w2662 w2674 w2720 _ _ w2770 w2837 w2904 w2971 w3038 w3105 w3172 w3240 w3308 w3375 w3442 w3510 w3521 w3560 w3600 w3640 w3680 w3720 w3778 w3813 w3849 w3882 w3952 w3985 w4018] -> w1240
      tunnel: [_ _ _ _ _ _ _ _ _ _ _ _ _ _ _ _ _ _ _ _ _ _ _ _ _ _ _ _ _ _ _ _ _ _ _ _ _ _ _ _ w3521 w3560 w3600 w3640 w3680 _ w3778 w3813 w3849 w3882 w3952 w3985 w4018] -> w1237
      event Timeout {
        n779 = event-data() -> ()  [unwired: 3 out]
      }
      event "停止": Value Change {
        n780 = event-data() -> ("NewVal"=w1247:bool)  [unwired: 5 out]
        n781 = stacked-sequence {
          tunnel: w1247 -> [w1266 _]
          tunnel: [w1266 _] -> w1246
          frame #0 {
            n782 = global read "配置文件全局.vi" "诊断标定读取地址"() -> (w1250:path)
            n783 = call <vilib>:"Application Directory.vi"() -> ("Application Directory"=w1260:path)
            n784 = property class="VI"("FP.State"=T24."Hidden" ("前面板窗口:状态")) -> (reference out=w1262:refnum<vi>, error out=w1261:errorcluster)  [unwired: 2 in]
            n785 = Build Path(base path=w1260, name or relative path="config.ini" ("名称或相对路径")) -> (appended path=w1258:path)
            n786 = call <vilib>:"Open Config Data.vi"("configuration file path"=w1258) -> ("error out"=w1255:errorcluster, "refnum"=w1257:T25)  [unwired: 8 in, 1 out]
            n787 = local write "停止"(TRUE ("停止")) -> ()
            n788 = property class="VI"(reference=w1262, error in=w1261, "Front Panel.Open"=FALSE ("前面板窗口:打开")) -> ()  [unwired: 2 out]
            n789 = call-poly <vilib>:"Write Key.vi"("section"="总信息", "error in (no error)"=w1255, "value"=w1250, "key"="诊断标定读取地址" ("section"), "refnum"=w1257) -> ("error out"=w1254:errorcluster, "refnum out"=w1253:T25)  [unwired: 4 in, 1 out]
            n790 = call <vilib>:"Close Config Data.vi"("error in (no error)"=w1254, "refnum"=w1253) -> ("error out"=w1252:errorcluster)  [unwired: 8 in, 1 out]
            n791 = call <vilib>:"Clear Errors.vi"("error in (no error)"=w1252) -> ()  [unwired: 6 in, 1 out]
          }
          frame #1 {
            n792 = disable-structure shown="禁用" {
              frame Disabled {
                n793 = local read "设备索引号"() -> (w1272:u16)
                n794 = local read "CAN卡类型"() -> (w1273:u32)
                n795 = local read "CAN端口"() -> (w1271:u16)
                n796 = Build Array(7) -> (w1268:i32[])
                n797 = call "transmit-8.6.vi"("can卡类型"=w1273, "设备索引号"=w1272, "CAN端口"=w1271, "ID"=418398080, "SendType"=u8 0, "Data"=w1268) -> ()  [unwired: 3 in, 11 out]
              }
              frame Enabled {
                w1280 = u8 0 items=["Normal", "Listen Only"] ("工作方式")
                w1279 = u8 1 items=["Dual Filter", "Single Filter"] ("滤波方式")
                n798 = local read "设备索引号"() -> (w1275:u16)
                n799 = local read "CAN卡类型"() -> (w1274:u32)
                n800 = local read "CAN端口"() -> (w1276:u16)
                n801 = call "CAN_Init-8.6.vi"("CAN卡类型"=w1274, "设备索引号"=w1275, "CAN端口"=w1276, "操作类型"=enum16{"初始化CAN", "关闭CAN"}."初始化CAN", "滤波方式"=w1279, "Accept Code"=u32 0, "簇"=T21 {"打开CAN"=FALSE, "初始化CAN"=TRUE, "开始CAN"=TRUE, "重启"=FALSE, "关闭CAN"=FALSE}, "Mask Code"=u32 4294967295 ("Accept Code"), "工作方式"=w1280, "是否滤波"=FALSE) -> ()  [unwired: 4 in, 6 out]
              }
            }
          }
        }
      }
      event Panel Close? {
        n802 = event-data() -> ()  [unwired: 5 out]
        n803 = stacked-sequence {
          tunnel: [w1299 _] -> w1286
          frame #0 {
            w1299 = TRUE ("前面板窗口:打开")
            n804 = global read "配置文件全局.vi" "诊断标定读取地址"() -> (w1288:path)
            n805 = call <vilib>:"Application Directory.vi"() -> ("Application Directory"=w1298:path)
            n806 = property class="VI"("FP.State"=T24."Hidden" ("前面板窗口:状态")) -> (reference out=w1301:refnum<vi>, error out=w1300:errorcluster)  [unwired: 2 in]
            n807 = Build Path(base path=w1298, name or relative path="config.ini" ("名称或相对路径")) -> (appended path=w1296:path)
            n808 = call <vilib>:"Open Config Data.vi"("configuration file path"=w1296) -> ("error out"=w1293:errorcluster, "refnum"=w1295:T25)  [unwired: 8 in, 1 out]
